vi "Open.vi"(8 "error in (no error)":errorcluster, 10 "File name (exclude extension)":string, 11 "Folder (create file inside this folder)":path) -> (0 "error out":errorcluster)   [LabVIEW 2018, in "text_file.lvlib"]
doc: "Opens (does not create) a text file (.txt extension)."
uses:
  text_file.lvlib
  private_data (library_variable).vi
panel:
  # "Development\ncontrols/indicators useful for development and testing, but which are not outputs of the VI"
  # "Input\nInputs to the VI"
  # "Output\nOutputs of the VI"
  # "Description\n\nBlank VI with error handling case. \n\nSummarize the use of this VI in this space."
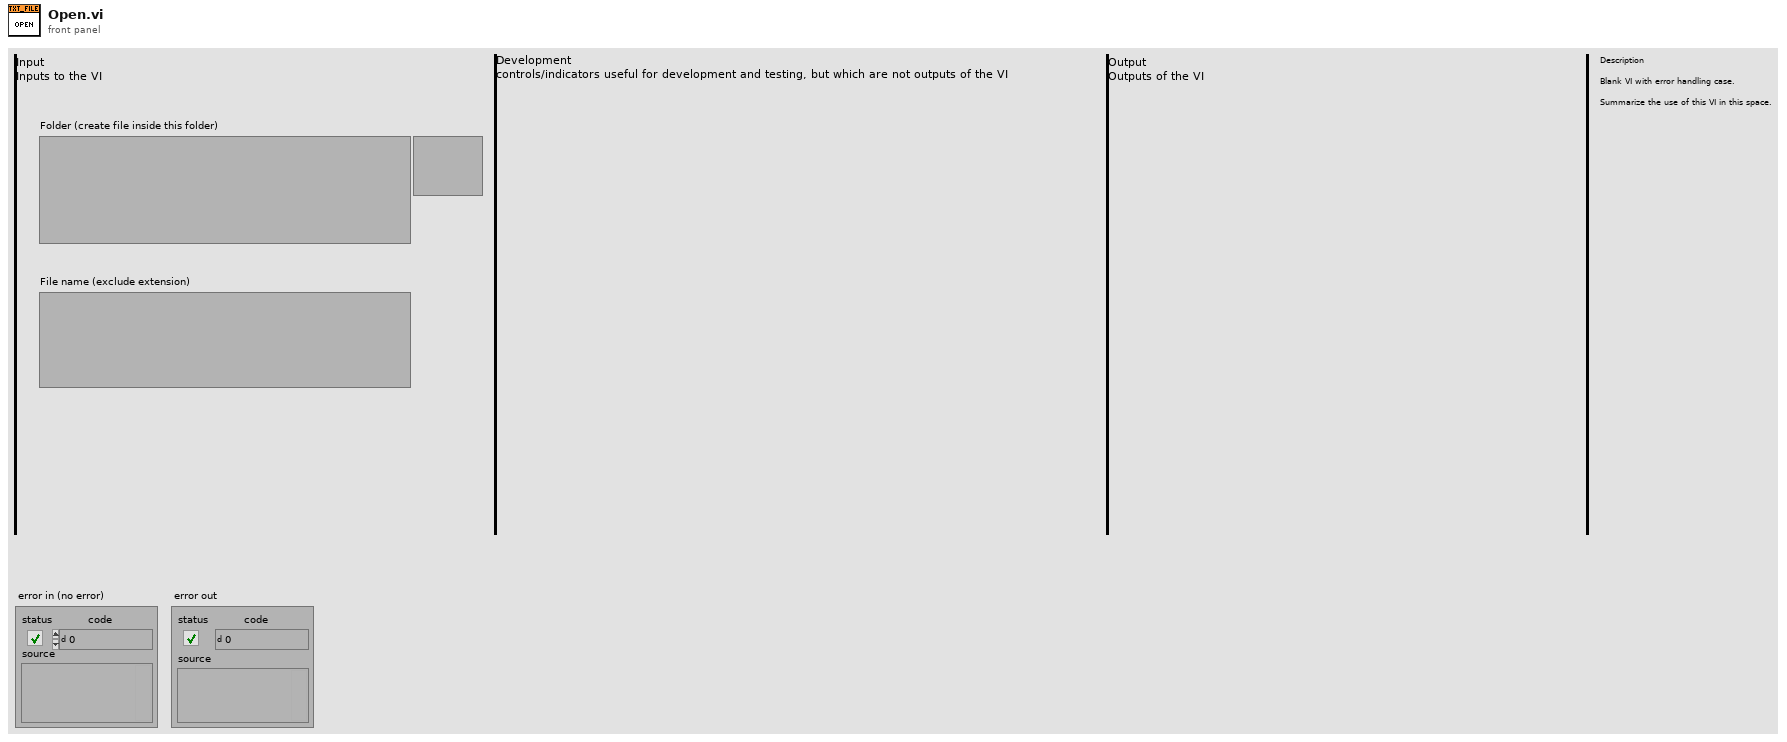
[diagram p1: front panel]
types:
  T1 = enum16{"open", "replace", "create", "open or create", "replace or create", "replace or create with confirmation"}
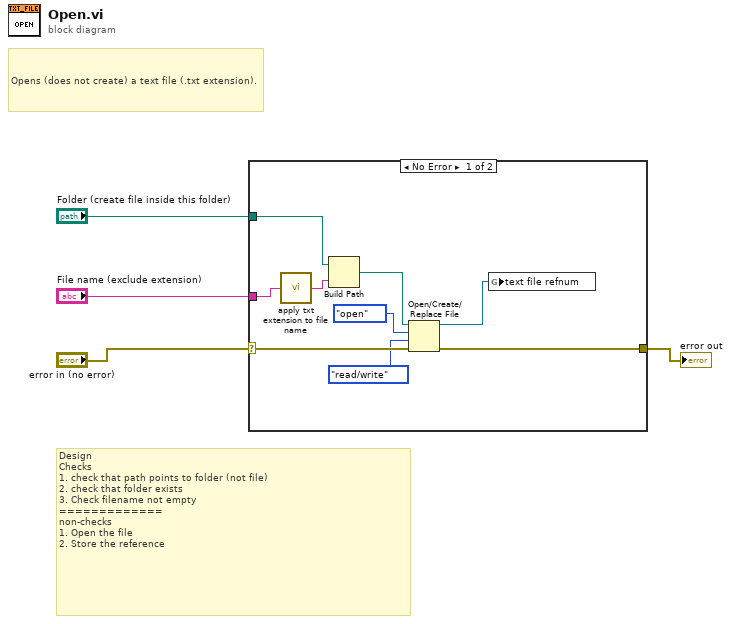
[diagram p0: block diagram]
diagram:
  # "Design\nChecks\n1. check that path points to folder (not file)\n2. check that folder exists\n3. Check filename not empty\n=============\nnon-checks\n1. Open the file\n2. Store the reference"
  # "Opens (does not create) a text file (.txt extension)."
  n1 = case shown="No Error" "error in (no error)" {
    selector: "error in (no error)" -> [w13 w14]
    tunnel: [w12 w14] -> w3
    tunnel: "Folder (create file inside this folder)" -> [w11 _]
    tunnel: "File name (exclude extension)" -> [w10 _]
    frame No Error {
      n2 = call "apply txt extension to file name.vi"("File name (excluding extension)"=w10) -> ("File name (with .txt extension)"=w5:string)
      n3 = Build Path(base path=w11, name or relative path=w5) -> (appended path=w9:path)
      n4 = Open/Create/Replace File(file path (use dialog)=w9, error in=w13, operation (0:open)=T1."open", access (0:read/write)=enum16{"read/write", "read-only", "write-only"}."read/write") -> (refnum out=w6:refnum<file>, error out=w12:errorcluster)  [unwired: 2 in, 1 out]
      n5 = global write "private_data (library_variable).vi" "text file refnum"(w6) -> ()
    }
    frame Error {
    }
  }
  "error out" <- w3
